vi "AttrMapToJson.vi"(8 "error in (no error)":errorcluster, 11 "AttrMap":T1) -> (0 "error out":errorcluster, 3 "Json":string)   [LabVIEW 2019, in "lv-apt-json-file.lvlib"]
uses:
  lv-apt-json-file.lvlib
  Typedef/Def-AttrMap.ctl
  <vilib>/addons/_JKI.lib/Serialization/JSON/JKI JSON Serialization.lvlib
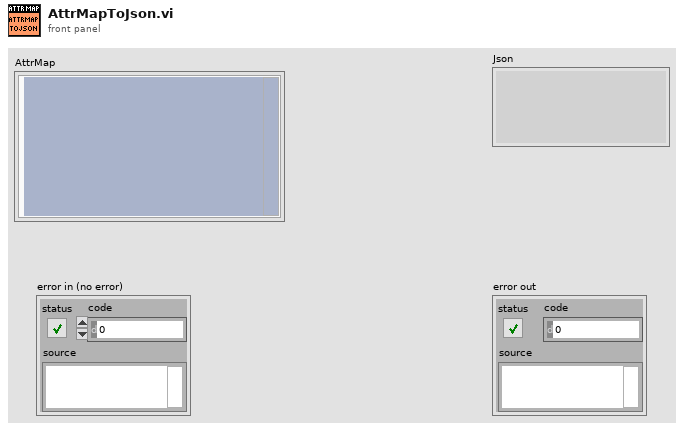
[diagram p1: front panel]
types:
  T1 = typedef "lv-apt-json-file.lvlib/Def-AttrMap.ctl" = cluster{"Map":variant}
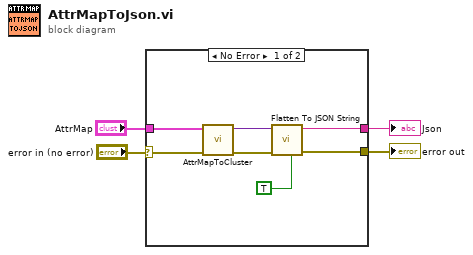
[diagram p0: block diagram]
diagram:
  n1 = case shown="No Error" "error in (no error)" {
    selector: "error in (no error)" -> [w11 w12]
    tunnel: "AttrMap" -> [w10 _]
    tunnel: [w9 _] -> w2
    tunnel: [w8 w12] -> w1
    frame No Error {
      n2 = call "AttrMapToCluster.vi"("error in (no error)"=w11, "AttrMap"=w10) -> ("error out"=w6:errorcluster, "Cluster"=w7:variant)  [unwired: 8 in]
      n3 = call <vilib>:"Flatten To JSON String.vi"("Enums As String (F)"=TRUE, "error in (no error)"=w6, "Variant"=w7) -> ("error out"=w8:errorcluster, "JSON String"=w9:string)  [unwired: 7 in]
    }
    frame Error {
    }
  }
  "Json" <- w2
  "error out" <- w1
